vi "FTP Move files.vi"(0 "File Management":T2, 1 "Unmanaged Files Queue":refnum<queue>, 3 "FTP Creds":T1 {"FTP Timeout (S)" min=0 max=300 step=1}, 4 "File output directories":T3={"Archive Location"=path "", "Archive Location 2"=path "<Not A Path>", "OutPut Path"=path "", "Directory(s) To Scan Files"=[]}, 5 "Unmanaged Files prior errors":errorcluster, 6 "Timing true or false to zip files":bool) -> (15 "Unmanaged Files Queue out":refnum<queue>, 16 "Unmanaged files queue error out":errorcluster, 19 "Log file write error condition":errorcluster)   [LabVIEW 2011]
uses:
  Controls/File Path directories.ctl
  Controls/File Management.ctl
  Controls/FTP Credintials.ctl
  <vilib>/Utility/sysdir.llb/System Directory Type.ctl
panel:
  # "File Handling Method"
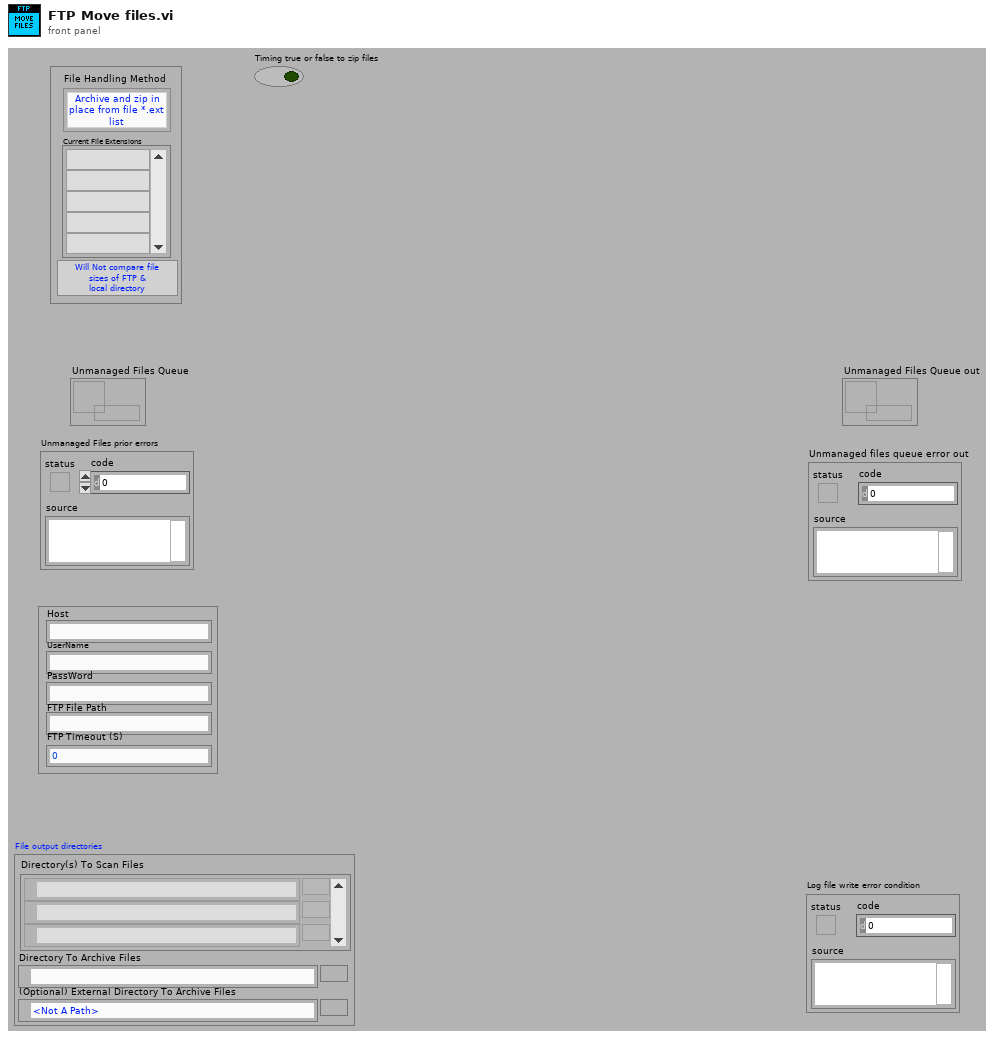
[diagram p1: front panel]
types:
  T1 = typedef "FTP Credintials.ctl" = cluster{"Host":string, "UserName":string, "PassWord":string, "FTP File Path":string, "FTP Timeout (S)":i32, "Active or Passive":bool, "ASCII or Binary":bool}
  T2 = typedef "File Management.ctl" = cluster{"Comp File Size":bool, "File Handle Method":enum16{"Archive and zip in place from file *.ext list", "Archive and zip ALL file Types to archive directory", "Archive and zip to archive directory from file *.ext list", "Perform no file management"}, "file extention list":string[]}
  T3 = typedef "File Path directories.ctl" = cluster{"Archive Location":path, "Archive Location 2":path, "OutPut Path":path, "Directory(s) To Scan Files":path[]}
  T4 = enum16{"Archive and zip in place from file *.ext list", "Archive and zip ALL file Types to archive directory", "Archive and zip to archive directory from file *.ext list", "Perform no file management"}
  T5 = typedef "System Directory Type.ctl" = i32
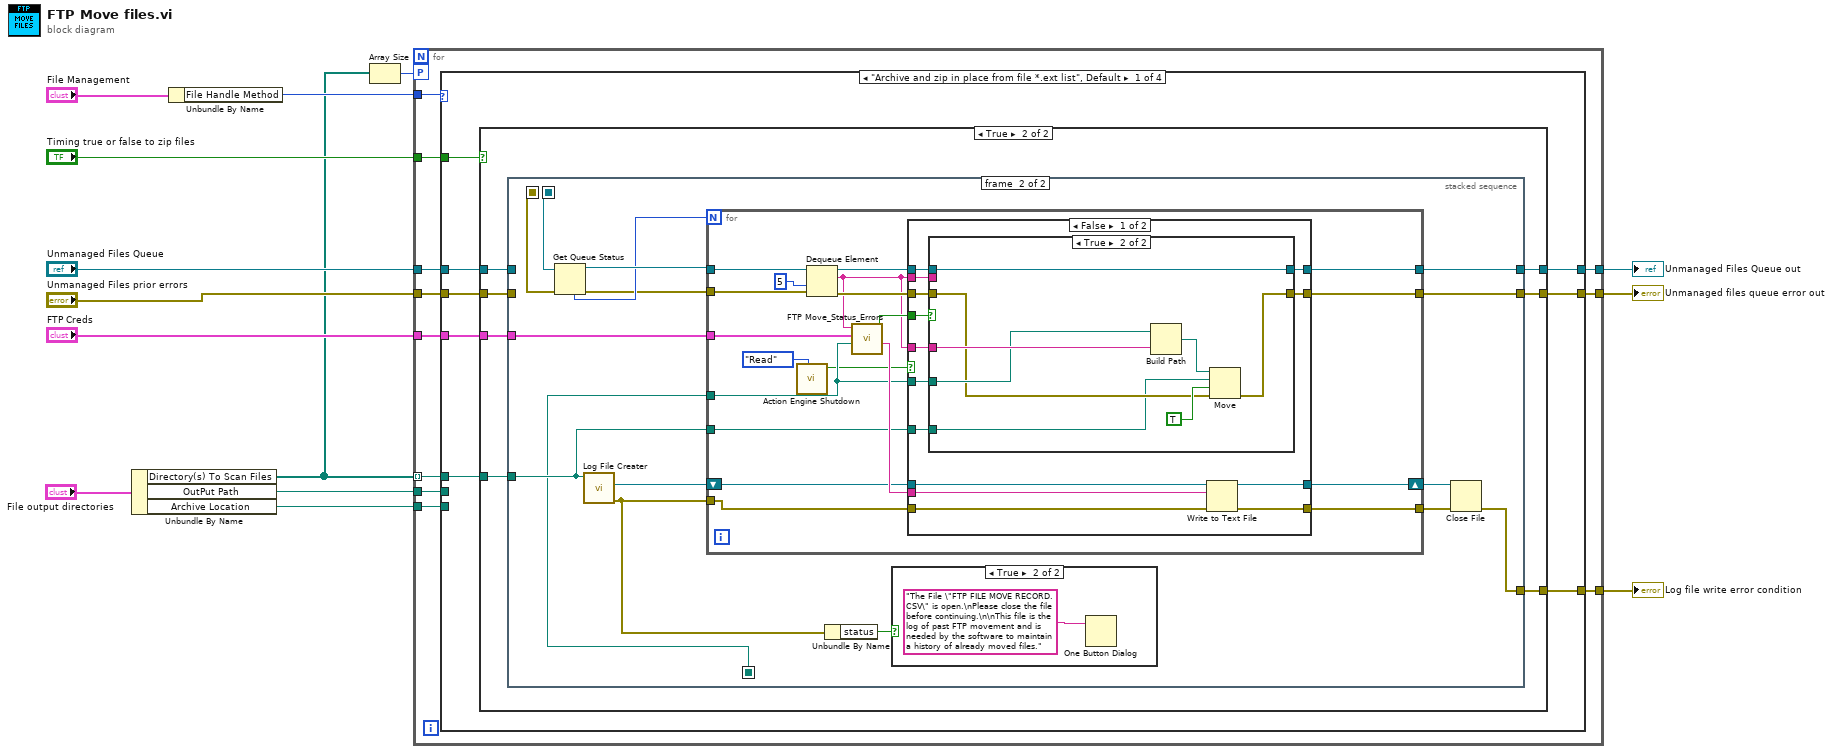
[diagram p0: block diagram]
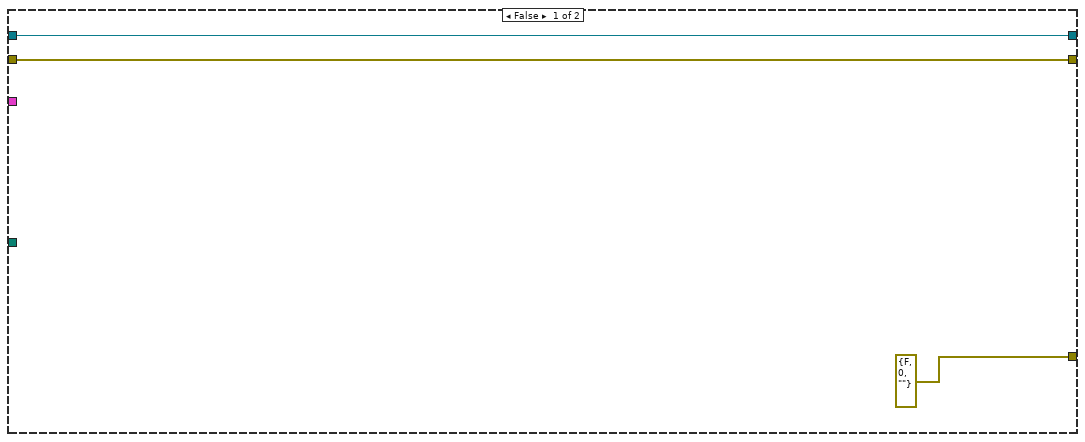
[diagram p2: hidden frame]
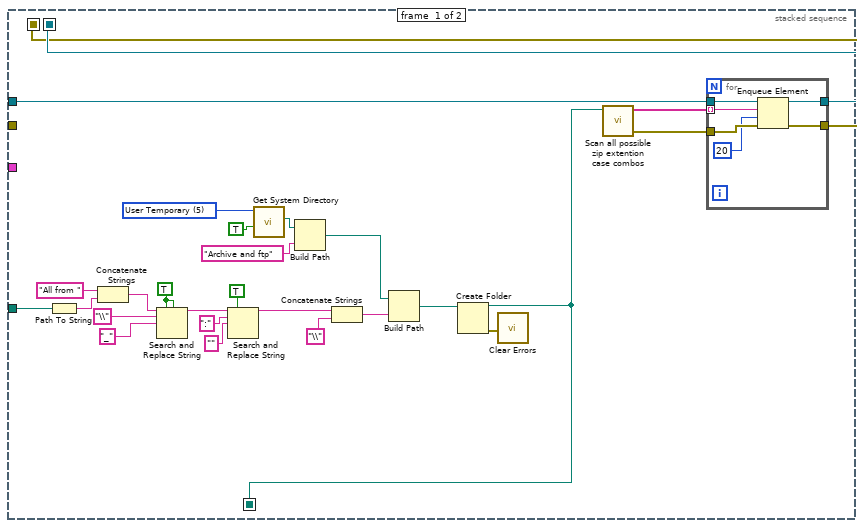
[diagram p3: hidden frame]
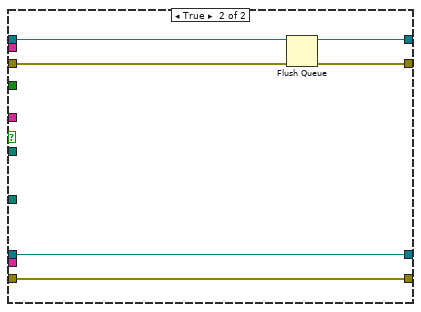
[diagram p6: hidden frame]
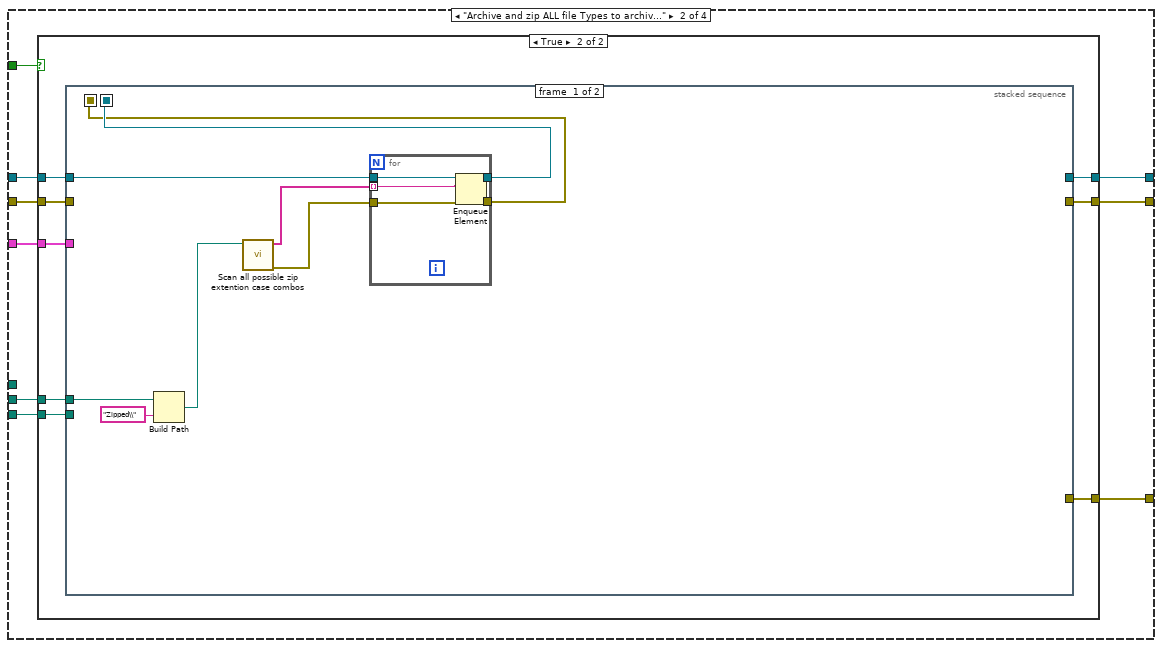
[diagram p7: hidden frame]
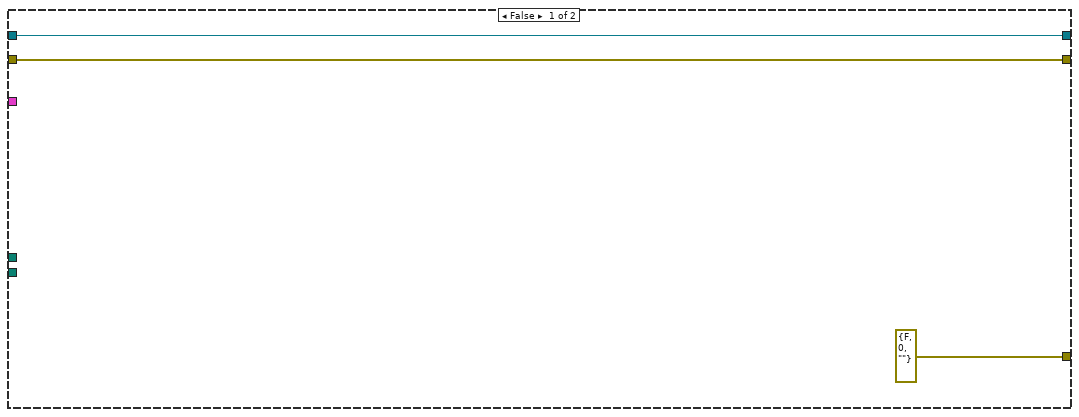
[diagram p8: hidden frame]
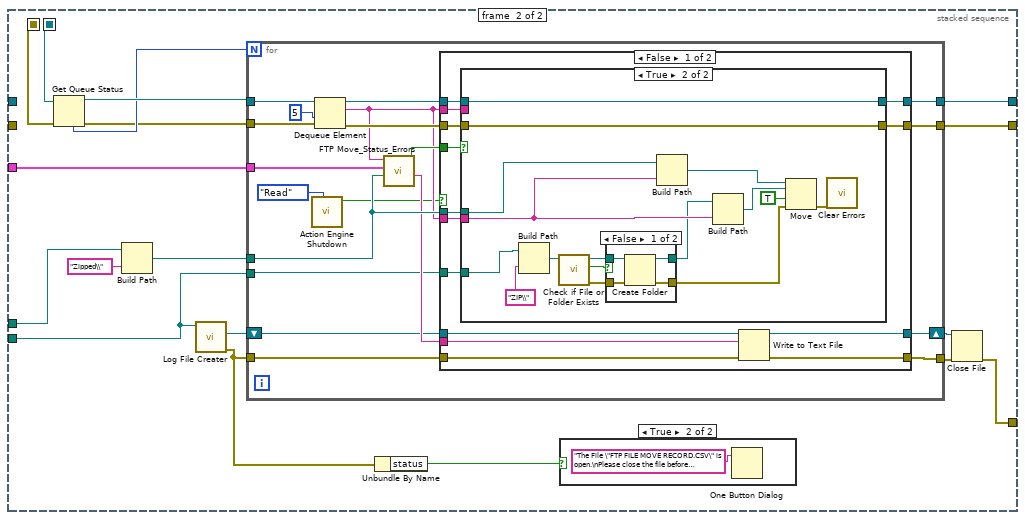
[diagram p9: hidden frame]
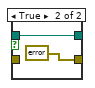
[diagram p12: hidden frame]
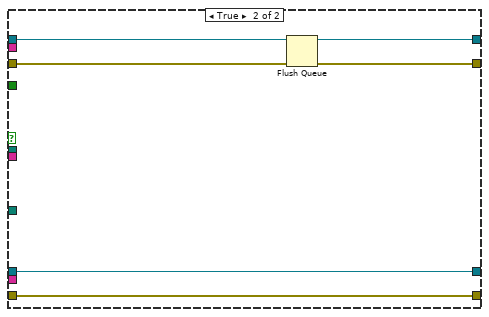
[diagram p13: hidden frame]
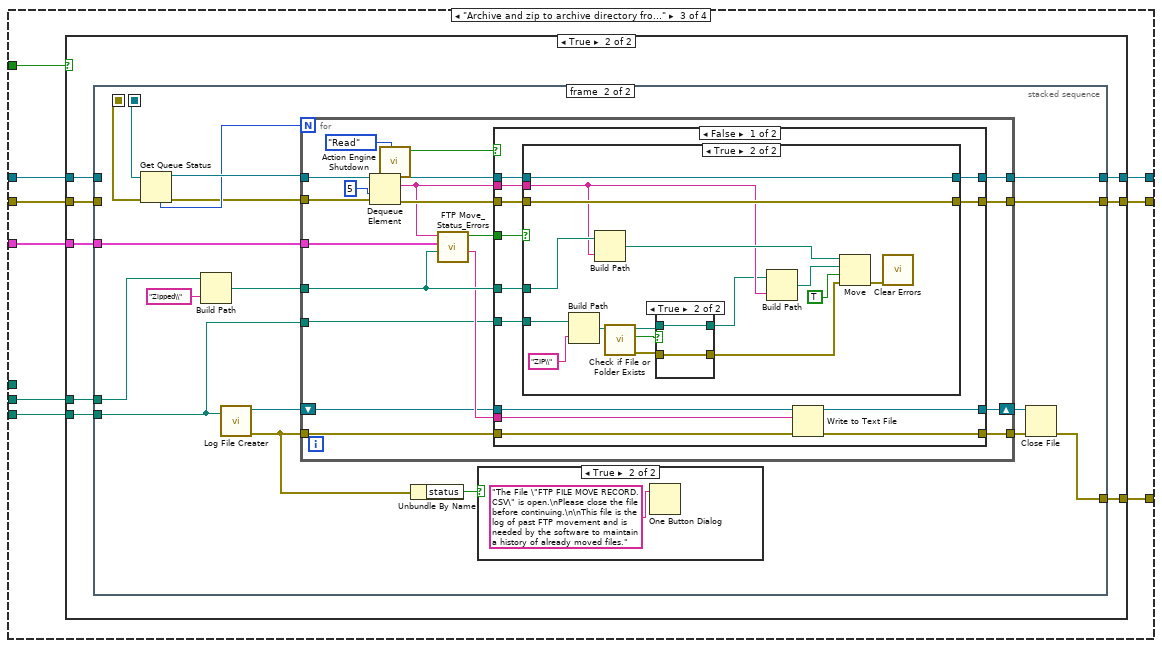
[diagram p14: hidden frame]
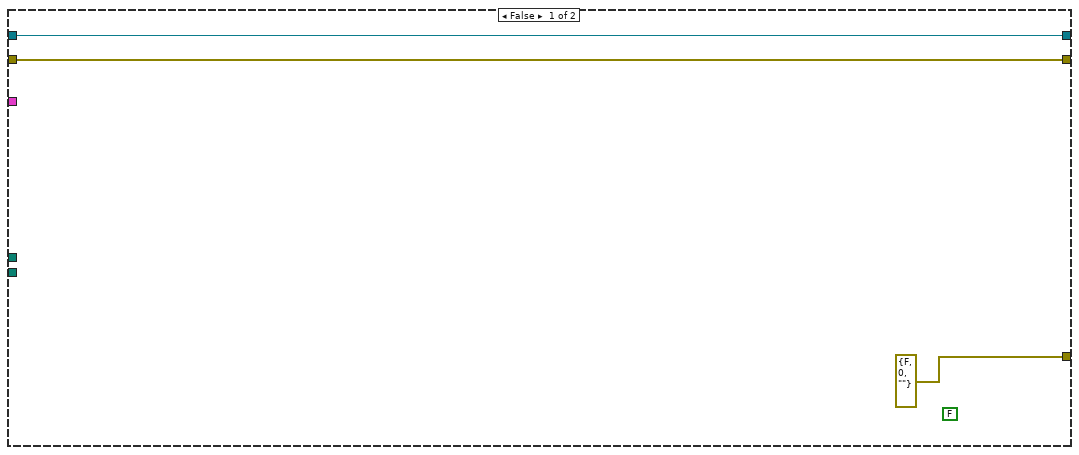
[diagram p15: hidden frame]
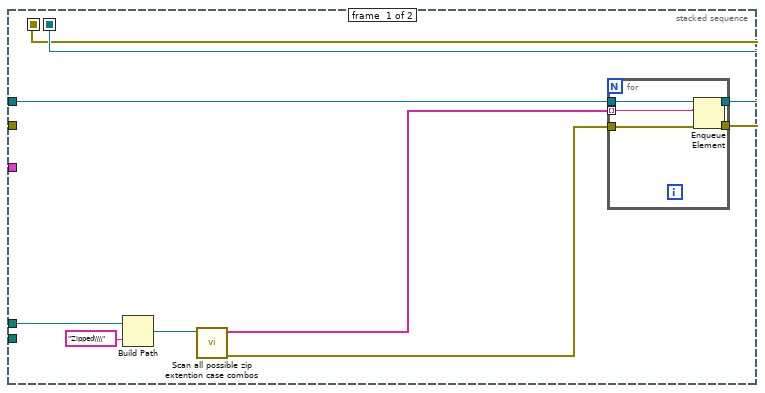
[diagram p16: hidden frame]
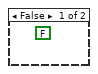
[diagram p17: hidden frame]
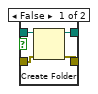
[diagram p19: hidden frame]
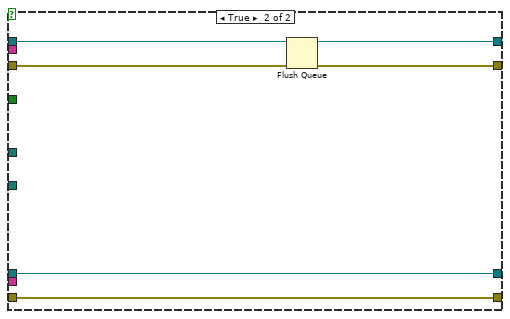
[diagram p20: hidden frame]
diagram:
  n1 = Unbundle By Name("File output directories") -> ("Directory(s) To Scan Files"=w1:path[], "OutPut Path"=w5:path, "Archive Location"=w4:path)
  n2 = Unbundle By Name("File Management") -> ("File Handle Method"=w6:T4)
  n3 = Array Size(array=w1) -> (size(s)=w2:i32)
  n4 = for {
    tunnel: "Unmanaged Files Queue" -> [w25]
    tunnel: "Unmanaged Files prior errors" -> [w24]
    tunnel: "Timing true or false to zip files" -> [w23]
    tunnel: [w22] -> w11
    tunnel: [w21] -> w10
    tunnel: [w20] -> w9
    tunnel: w6 -> [w19]
    tunnel: w5 -> [w18]
    tunnel: w4 -> [w17]
    tunnel: "FTP Creds" -> [w16]
    tunnel: w1 -> [w15] mode=indexing
    workers-P: w2 -> [_]
    n5 = case shown="\"Archive and zip in place from file *.ext list\", Default" w19 {
      tunnel: w25 -> [w32 w151 w265 w374]
      tunnel: w24 -> [w31 w150 w264 w373]
      tunnel: w16 -> [w30 w149 w263 _]
      tunnel: w18 -> [_ w148 w262 _]
      tunnel: w23 -> [w33 w147 w266 _]
      tunnel: [w28 w146 w260 w374] -> w22
      tunnel: [w27 w145 w259 w373] -> w21
      tunnel: [w26 w144 w258 errorcluster {"status"=FALSE, "code"=0, "source"=""} ("error out")] -> w20
      tunnel: w17 -> [_ w143 w261 _]
      tunnel: w15 -> [w29 _ _ _]
      frame "Archive and zip in place from file *.ext list", Default {
        n6 = case shown="True" w33 {
          tunnel: w32 -> [w36 w43]
          tunnel: [w36 w42] -> w28
          tunnel: w31 -> [w35 w41]
          tunnel: [w35 w40] -> w27
          tunnel: [errorcluster {"status"=FALSE, "code"=0, "source"=""} ("error out") w37] -> w26
          tunnel: w30 -> [_ w39]
          tunnel: w29 -> [_ w38]
          frame False {
          }
          frame True {
            n7 = stacked-sequence {
              seq-local: [w69 _] -> [_ w91]
              seq-local: [w68 _] -> [_ w85]
              seq-local: [w46 _] -> [_ w78]
              tunnel: w43 -> [w70 _]
              tunnel: [_ w92] -> w42
              tunnel: w41 -> [_ _]
              tunnel: [_ w87] -> w40
              tunnel: w39 -> [_ w86]
              tunnel: w38 -> [w47 w79]
              tunnel: [_ w82] -> w37
              frame #0 {
                w58 = TRUE ("replace all? (F)")
                w51 = T5 5 items=["User Home"=0, "User Desktop"=1, "User Documents"=2, "User Application Data"=3, "User Preferences"=4, "User Temporary"=5, "Public Documents"=6, "Public Application Data"=7, "Public Preferences"=8, "Public Cache"=13, "System Core Libraries"=9, "System Installed Libraries"=10, "Application Files"=11, "Boot Volume Root"=12] ("system directory type")
                n8 = Path To String(path=w47) -> (string=w54:string)
                n9 = Concatenate Strings("All from " ("name or relative path"), w54) -> (w55:string)
                n10 = Search and Replace String(replace all?=w58, case sensitive?=w58, input string=w55, search string="\\" ("replace string (\"\")"), replace string="_" ("replace string (\"\")")) -> (result string=w61:string)  [unwired: 3 in, 3 out]
                n11 = Search and Replace String(replace all?=TRUE ("replace all? (F)"), input string=w61, search string=":" ("replace string (\"\")"), replace string="" ("replace string (\"\")")) -> (result string=w64:string)  [unwired: 4 in, 3 out]
                n12 = call <vilib>:"Get System Directory.vi"("create directory if not found? (F)"=TRUE, "system directory type"=w51) -> ("system directory"=w49:path)  [unwired: 9 in]
                n13 = Build Path(base path=w49, name or relative path="Archive and ftp") -> (appended path=w63:path)
                n14 = Concatenate Strings(w64, "\\" ("replace string (\"\")")) -> (w66:string)
                n15 = Build Path(base path=w63, name or relative path=w66) -> (appended path=w67:path)
                n16 = Create Folder(path (use dialog)=w67) -> (created path=w46:path, error out=w52:errorcluster)  [unwired: 2 in, 1 out]
                n17 = call <vilib>:"Clear Errors.vi"("error in (no error)"=w52) -> ()  [unwired: 6 in, 1 out]
                n18 = call "Scan all possible zip extention case combos.vi"("Path containing Zipped files"=w46) -> ("error out"=w44:errorcluster, "Zipped Files List"=w45:string[])  [unwired: 9 in]
                n19 = for {
                  tunnel: w70 -> [w76]
                  tunnel: [w75] -> w68
                  tunnel: [w74] -> w69
                  tunnel: w45 -> [w73] mode=indexing
                  tunnel: w44 -> [w72]
                  n20 = Enqueue Element(queue=w76, element=w73, timeout in ms (-1)=20, error in (no error)=w72) -> (queue out=w74:refnum<queue>, error out=w75:errorcluster)  [unwired: 1 out]
                }
              }
              frame #1 {
                n21 = Get Queue Status(queue=w91, error in (no error)=w85) -> (queue out=w90:refnum<queue>, error out=w88:errorcluster, # elements in queue=w89:i32)  [unwired: 1 in, 5 out]
                n22 = call "Log File Creater.vi"("FTP log file path"=w79) -> ("all condition error"=w77:errorcluster, "File Refnum"=w81:refnum<file>)  [unwired: 8 in, 1 out]
                n23 = for {
                  N: w89 -> [_]
                  tunnel: w90 -> [w105]
                  tunnel: [w111] -> w92
                  tunnel: w88 -> [w104]
                  tunnel: [w108] -> w87
                  tunnel: w86 -> [w107]
                  tunnel: w79 -> [w101]
                  tunnel: w78 -> [w100]
                  tunnel: [w98] -> w83
                  tunnel: w77 -> [w96]
                  shift-right: [w99] -> w80
                  shift-left: w81 -> [w97]
                  n24 = call "Action Engine Shutdown.vi"("Shutdown"=enum16{"Write", "Read"}."Read") -> ("Shutdown"=w94:bool)  [unwired: 9 in, 1 out]
                  n25 = Dequeue Element(queue=w105, timeout in ms (-1)=5, error in (no error)=w104) -> (queue out=w112:refnum<queue>, element=w102:string, error out=w109:errorcluster)  [unwired: 1 out]
                  n26 = call "FTP Move_Status_Errors.vi"("Dir of file to FTP"=w100, "FTP input cluster"=w107, "File to Move"=w102) -> ("concatenated string of Error"=w103:string, "FTP completed (true = good)"=w106:bool)  [unwired: 7 in]
                  n27 = case shown="False" w94 {
                    tunnel: [w126 w138] -> w99
                    tunnel: [w125 w137] -> w98
                    tunnel: w112 -> [w124 w142]
                    tunnel: [w123 w141] -> w111
                    tunnel: w109 -> [w122 w140]
                    tunnel: [w121 w139] -> w108
                    tunnel: w103 -> [w120 _]
                    tunnel: w106 -> [w119 _]
                    tunnel: w102 -> [w118 _]
                    tunnel: w101 -> [w117 _]
                    tunnel: w102 -> [w116 _]
                    tunnel: w97 -> [w115 w138]
                    tunnel: w96 -> [w114 w137]
                    tunnel: w100 -> [w113 _]
                    frame False {
                      n28 = case shown="True" w119 {
                        tunnel: w124 -> [w128 w136]
                        tunnel: w118 -> [_ _]
                        tunnel: [w128 w136] -> w123
                        tunnel: w122 -> [w127 w130]
                        tunnel: [w127 w133] -> w121
                        tunnel: w117 -> [_ w129]
                        tunnel: w116 -> [_ w135]
                        tunnel: w113 -> [_ w131]
                        frame False {
                          # "If Error occurs in ftp then leave element alone\nand it will be requeued next time process runs."
                        }
                        frame True {
                          n29 = Build Path(base path=w131, name or relative path=w135) -> (appended path=w134:path)
                          n30 = Move(source path=w134, error in=w130, 9:TRUE ("overwrite (F)"), 10:w129) -> (error out=w133:errorcluster)  [unwired: 1 in, 2 out]
                        }
                      }
                      n31 = Write to Text File(file (use dialog)=w115, text=w120, error in=w114) -> (refnum out=w126:refnum<file>, error out=w125:errorcluster)  [unwired: 1 in, 1 out]
                    }
                    frame True {
                      n32 = Flush Queue(queue=w142, error in (no error)=w140) -> (queue out=w141:refnum<queue>, error out=w139:errorcluster)  [unwired: 1 out]
                    }
                  }
                }
                n33 = Unbundle By Name(w77) -> ("status"=w84:bool)
                n34 = case shown="True" w84 {
                  frame False {
                  }
                  frame True {
                    n35 = One Button Dialog(message="The File \"FTP FILE MOVE RECORD.CSV\" is open.\nPlease close the file before continuing.\n\nThis file is the log of past FTP movement and is needed by the software to maintain a history of already moved files.") -> ()  [unwired: 1 in, 1 out]
                  }
                }
                n36 = Close File(refnum=w80, error in=w83) -> (error out=w82:errorcluster)  [unwired: 1 out]
              }
            }
          }
        }
      }
      frame "Archive and zip ALL file Types to archive directory" {
        n37 = case shown="True" w147 {
          tunnel: w151 -> [w154 w162]
          tunnel: [w154 w161] -> w146
          tunnel: w150 -> [w153 w160]
          tunnel: [w153 w159] -> w145
          tunnel: [errorcluster {"status"=FALSE, "code"=0, "source"=""} ("error out") w155] -> w144
          tunnel: w149 -> [_ w158]
          tunnel: w148 -> [_ w157]
          tunnel: w143 -> [_ w156]
          frame False {
          }
          frame True {
            n38 = stacked-sequence {
              seq-local: [w169 _] -> [_ w192]
              seq-local: [w168 _] -> [_ w186]
              tunnel: w162 -> [w170 _]
              tunnel: [_ w193] -> w161
              tunnel: w160 -> [_ _]
              tunnel: [_ w188] -> w159
              tunnel: w158 -> [_ w187]
              tunnel: w157 -> [w167 w177]
              tunnel: w156 -> [_ w180]
              tunnel: [_ w182] -> w155
              frame #0 {
                n39 = Build Path(base path=w167, name or relative path="Zipped\\") -> (appended path=w165:path)
                n40 = call "Scan all possible zip extention case combos.vi"("Path containing Zipped files"=w165) -> ("error out"=w163:errorcluster, "Zipped Files List"=w164:string[])  [unwired: 9 in]
                n41 = for {
                  tunnel: w170 -> [w175]
                  tunnel: [w174] -> w168
                  tunnel: [w173] -> w169
                  tunnel: w164 -> [w172] mode=indexing
                  tunnel: w163 -> [w171]
                  n42 = Enqueue Element(queue=w175, element=w172, error in (no error)=w171) -> (queue out=w173:refnum<queue>, error out=w174:errorcluster)  [unwired: 1 in, 1 out]
                }
              }
              frame #1 {
                n43 = Get Queue Status(queue=w192, error in (no error)=w186) -> (queue out=w191:refnum<queue>, error out=w189:errorcluster, # elements in queue=w190:i32)  [unwired: 1 in, 5 out]
                n44 = Build Path(base path=w177, name or relative path="Zipped\\") -> (appended path=w178:path)
                n45 = call "Log File Creater.vi"("FTP log file path"=w180) -> ("all condition error"=w176:errorcluster, "File Refnum"=w181:refnum<file>)  [unwired: 8 in, 1 out]
                n46 = for {
                  N: w190 -> [_]
                  tunnel: w191 -> [w206]
                  tunnel: [w212] -> w193
                  tunnel: w189 -> [w205]
                  tunnel: [w209] -> w188
                  tunnel: w187 -> [w208]
                  tunnel: w178 -> [w204]
                  tunnel: [w200] -> w183
                  tunnel: w176 -> [w198]
                  tunnel: w180 -> [w197]
                  shift-right: [w201] -> w184
                  shift-left: w181 -> [w199]
                  n47 = call "Action Engine Shutdown.vi"("Shutdown"=enum16{"Write", "Read"}."Read") -> ("Shutdown"=w195:bool)  [unwired: 9 in, 1 out]
                  n48 = Dequeue Element(queue=w206, timeout in ms (-1)=5, error in (no error)=w205) -> (queue out=w213:refnum<queue>, element=w202:string, error out=w210:errorcluster)  [unwired: 1 out]
                  n49 = call "FTP Move_Status_Errors.vi"("Dir of file to FTP"=w204, "FTP input cluster"=w208, "File to Move"=w202) -> ("concatenated string of Error"=w203:string, "FTP completed (true = good)"=w207:bool)  [unwired: 7 in]
                  n50 = case shown="False" w195 {
                    tunnel: [w227 w253] -> w201
                    tunnel: [w226 w252] -> w200
                    tunnel: w213 -> [w225 w257]
                    tunnel: [w224 w256] -> w212
                    tunnel: w210 -> [w223 w255]
                    tunnel: [w222 w254] -> w209
                    tunnel: w203 -> [w221 _]
                    tunnel: w207 -> [w220 _]
                    tunnel: w202 -> [w219 _]
                    tunnel: w204 -> [w218 _]
                    tunnel: w202 -> [w217 _]
                    tunnel: w199 -> [w216 w253]
                    tunnel: w198 -> [w215 w252]
                    tunnel: w197 -> [w214 _]
                    frame False {
                      n51 = case shown="True" w220 {
                        tunnel: w225 -> [w229 w245]
                        tunnel: w219 -> [_ _]
                        tunnel: [w229 w245] -> w224
                        tunnel: w223 -> [w228 w244]
                        tunnel: [w228 w244] -> w222
                        tunnel: w218 -> [_ w243]
                        tunnel: w217 -> [_ w240]
                        tunnel: w214 -> [_ w233]
                        frame False {
                        }
                        frame True {
                          n52 = Build Path(base path=w233, name or relative path="ZIP\\") -> (appended path=w236:path)
                          n53 = call <vilib>:"Check if File or Folder Exists.vi"("path"=w236) -> ("error out"=w230:errorcluster, "file or folder exists?"=w237:bool, "dup path"=w238:path)  [unwired: 8 in]
                          n54 = case shown="False" w237 {
                            tunnel: w238 -> [w249 w251]
                            tunnel: [w248 w251] -> w234
                            tunnel: [w247 errorcluster {"status"=FALSE, "code"=0, "source"=""} ("error out")] -> w232
                            tunnel: w230 -> [w246 _]
                            frame False {
                              n55 = Create Folder(path (use dialog)=w249, error in=w246) -> (created path=w248:path, error out=w247:errorcluster)  [unwired: 1 in, 1 out]
                            }
                            frame True {
                            }
                          }
                          n56 = Build Path(base path=w243, name or relative path=w240) -> (appended path=w242:path)
                          n57 = Build Path(base path=w234, name or relative path=w240) -> (appended path=w241:path)
                          n58 = Move(source path=w242, error in=w232, 9:TRUE ("overwrite (F)"), 10:w241) -> (error out=w231:errorcluster)  [unwired: 1 in, 2 out]
                          n59 = call <vilib>:"Clear Errors.vi"("error in (no error)"=w231) -> ()  [unwired: 6 in, 1 out]
                        }
                      }
                      n60 = Write to Text File(file (use dialog)=w216, text=w221, error in=w215) -> (refnum out=w227:refnum<file>, error out=w226:errorcluster)  [unwired: 1 in, 1 out]
                    }
                    frame True {
                      n61 = Flush Queue(queue=w257, error in (no error)=w255) -> (queue out=w256:refnum<queue>, error out=w254:errorcluster)  [unwired: 1 out]
                    }
                  }
                }
                n62 = Unbundle By Name(w176) -> ("status"=w185:bool)
                n63 = case shown="True" w185 {
                  frame False {
                  }
                  frame True {
                    n64 = One Button Dialog(message="The File \"FTP FILE MOVE RECORD.CSV\" is open.\nPlease close the file before continuing.\n\nThis file is the log of past FTP movement and is needed by the software to maintain a history of already moved files.") -> ()  [unwired: 1 in, 1 out]
                  }
                }
                n65 = Close File(refnum=w184, error in=w183) -> (error out=w182:errorcluster)  [unwired: 1 out]
              }
            }
          }
        }
      }
      frame "Archive and zip to archive directory from file *.ext list" {
        n66 = case shown="True" w266 {
          tunnel: w265 -> [w269 w277]
          tunnel: [w269 w276] -> w260
          tunnel: w264 -> [w268 w275]
          tunnel: [w268 w274] -> w259
          tunnel: [errorcluster {"status"=FALSE, "code"=0, "source"=""} ("error out") w273] -> w258
          tunnel: w263 -> [_ w272]
          tunnel: w262 -> [_ w271]
          tunnel: w261 -> [_ w270]
          frame False {
            (unwired) FALSE
          }
          frame True {
            n67 = stacked-sequence {
              seq-local: [w284 _] -> [_ w307]
              seq-local: [w281 _] -> [_ w301]
              tunnel: w277 -> [w285 _]
              tunnel: [_ w308] -> w276
              tunnel: w275 -> [_ _]
              tunnel: [_ w303] -> w274
              tunnel: [_ w297] -> w273
              tunnel: w272 -> [_ w302]
              tunnel: w271 -> [w280 w292]
              tunnel: w270 -> [_ w295]
              frame #0 {
                n68 = Build Path(base path=w280, name or relative path="Zipped\\\\") -> (appended path=w279:path)
                n69 = call "Scan all possible zip extention case combos.vi"("Path containing Zipped files"=w279) -> ("error out"=w282:errorcluster, "Zipped Files List"=w283:string[])  [unwired: 9 in]
                n70 = for {
                  tunnel: w285 -> [w290]
                  tunnel: [w289] -> w281
                  tunnel: [w288] -> w284
                  tunnel: w283 -> [w287] mode=indexing
                  tunnel: w282 -> [w286]
                  n71 = Enqueue Element(queue=w290, element=w287, error in (no error)=w286) -> (queue out=w288:refnum<queue>, error out=w289:errorcluster)  [unwired: 1 in, 1 out]
                }
              }
              frame #1 {
                n72 = Get Queue Status(queue=w307, error in (no error)=w301) -> (queue out=w306:refnum<queue>, error out=w304:errorcluster, # elements in queue=w305:i32)  [unwired: 1 in, 5 out]
                n73 = Build Path(base path=w292, name or relative path="Zipped\\") -> (appended path=w293:path)
                n74 = call "Log File Creater.vi"("FTP log file path"=w295) -> ("all condition error"=w291:errorcluster, "File Refnum"=w296:refnum<file>)  [unwired: 8 in, 1 out]
                n75 = for {
                  N: w305 -> [_]
                  tunnel: w306 -> [w321]
                  tunnel: [w327] -> w308
                  tunnel: [w315] -> w298
                  tunnel: w304 -> [w320]
                  tunnel: [w324] -> w303
                  tunnel: w302 -> [w323]
                  tunnel: w293 -> [w319]
                  tunnel: w295 -> [w314]
                  tunnel: w291 -> [w312]
                  shift-right: [w316] -> w299
                  shift-left: w296 -> [w313]
                  n76 = Dequeue Element(queue=w321, timeout in ms (-1)=5, error in (no error)=w320) -> (queue out=w328:refnum<queue>, element=w317:string, error out=w325:errorcluster)  [unwired: 1 out]
                  n77 = call "Action Engine Shutdown.vi"("Shutdown"=enum16{"Write", "Read"}."Read") -> ("Shutdown"=w310:bool)  [unwired: 9 in, 1 out]
                  n78 = call "FTP Move_Status_Errors.vi"("Dir of file to FTP"=w319, "FTP input cluster"=w323, "File to Move"=w317) -> ("concatenated string of Error"=w318:string, "FTP completed (true = good)"=w322:bool)  [unwired: 7 in]
                  n79 = case shown="False" w310 {
                    tunnel: [w341 w367] -> w316
                    tunnel: [w340 w366] -> w315
                    tunnel: w328 -> [w339 w371]
                    tunnel: [w338 w370] -> w327
                    tunnel: w325 -> [w337 w369]
                    tunnel: [w336 w368] -> w324
                    tunnel: w318 -> [w335 _]
                    tunnel: w322 -> [w334 _]
                    tunnel: w319 -> [w333 _]
                    tunnel: w317 -> [w332 _]
                    tunnel: w313 -> [w331 w367]
                    tunnel: w312 -> [w330 w366]
                    tunnel: w314 -> [w329 _]
                    frame False {
                      n80 = case shown="True" w334 {
                        tunnel: w339 -> [w343 w359]
                        tunnel: [w343 w359] -> w338
                        tunnel: w337 -> [w342 w358]
                        tunnel: [w342 w358] -> w336
                        tunnel: w333 -> [_ w357]
                        tunnel: w332 -> [_ w354]
                        tunnel: w329 -> [_ w347]
                        frame False {
                        }
                        frame True {
                          n81 = Build Path(base path=w347, name or relative path="ZIP\\") -> (appended path=w350:path)
                          n82 = Build Path(base path=w357, name or relative path=w354) -> (appended path=w356:path)
                          n83 = call <vilib>:"Check if File or Folder Exists.vi"("path"=w350) -> ("error out"=w346:errorcluster, "file or folder exists?"=w351:bool, "dup path"=w352:path)  [unwired: 8 in]
                          n84 = case shown="True" w351 {
                            tunnel: w352 -> [w363 w365]
                            tunnel: [w362 w365] -> w348
                            tunnel: w346 -> [w361 w364]
                            tunnel: [w360 w364] -> w345
                            frame False {
                              n85 = Create Folder(path (use dialog)=w363, error in=w361) -> (created path=w362:path, error out=w360:errorcluster)  [unwired: 1 in, 1 out]
                            }
                            frame True {
                            }
                          }
                          n86 = Build Path(base path=w348, name or relative path=w354) -> (appended path=w355:path)
                          n87 = Move(source path=w356, error in=w345, 9:TRUE ("overwrite (F)"), 10:w355) -> (error out=w344:errorcluster)  [unwired: 1 in, 2 out]
                          n88 = call <vilib>:"Clear Errors.vi"("error in (no error)"=w344) -> ()  [unwired: 6 in, 1 out]
                        }
                      }
                      n89 = Write to Text File(file (use dialog)=w331, text=w335, error in=w330) -> (refnum out=w341:refnum<file>, error out=w340:errorcluster)  [unwired: 1 in, 1 out]
                    }
                    frame True {
                      n90 = Flush Queue(queue=w371, error in (no error)=w369) -> (queue out=w370:refnum<queue>, error out=w368:errorcluster)  [unwired: 1 out]
                    }
                  }
                }
                n91 = Unbundle By Name(w291) -> ("status"=w300:bool)
                n92 = case shown="True" w300 {
                  frame False {
                    (unwired) FALSE
                  }
                  frame True {
                    n93 = One Button Dialog(message="The File \"FTP FILE MOVE RECORD.CSV\" is open.\nPlease close the file before continuing.\n\nThis file is the log of past FTP movement and is needed by the software to maintain a history of already moved files.") -> ()  [unwired: 1 in, 1 out]
                  }
                }
                n94 = Close File(refnum=w299, error in=w298) -> (error out=w297:errorcluster)  [unwired: 1 out]
              }
            }
          }
        }
      }
      frame "Perform no file management" {
      }
    }
  }
  "Unmanaged Files Queue out" <- w11
  "Unmanaged files queue error out" <- w10
  "Log file write error condition" <- w9
